vi "De-Initialize.vi"(8 "error in (no error)":errorcluster, 11 "Device in":refnum<class "RS232_Device.lvclass">) -> (0 "error out":errorcluster, 3 "Device out":refnum<class "RS232_Device.lvclass">)   [LabVIEW 2023, in "RS232_Device.lvclass"]
uses:
  RS232_Device.lvclass
  RS232_Device.lvclass/RS232_Device.ctl
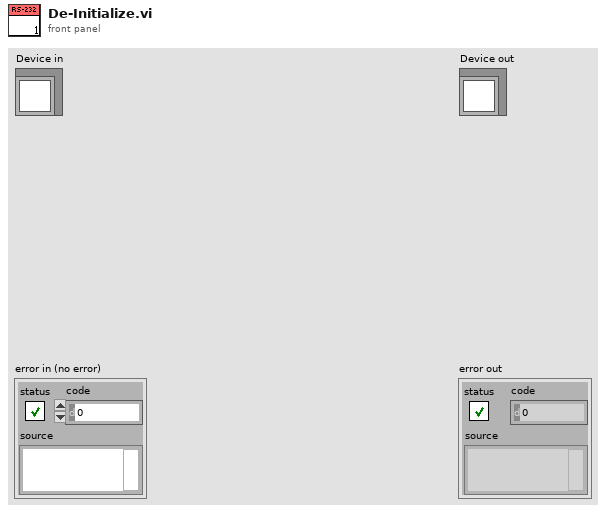
[diagram p1: front panel]
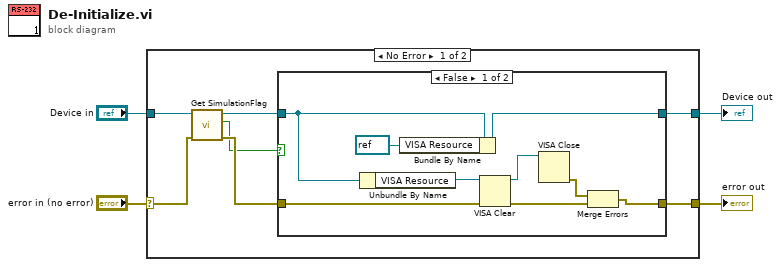
[diagram p0: block diagram]
diagram:
  n1 = case shown="No Error" "error in (no error)" {
    selector: "error in (no error)" -> [w7 w24]
    tunnel: [w11 w24] -> w3
    tunnel: [w10 w23] -> w1
    tunnel: "Device in" -> [w8 w23]
    frame No Error {
      n2 = call-dynamic "Get SimulationFlag.vi"("error in (no error)"=w7, "Device in"=w8) -> ("error out"=w6:errorcluster, "Simulation?"=w5:bool, "Device out"=w9:refnum<class "RS232_Device.lvclass">)  [unwired: 7 in]
      n3 = case shown="False" w5 {
        tunnel: w9 -> [w20 w22]
        tunnel: w6 -> [w15 w21]
        tunnel: [w12 w21] -> w11
        tunnel: [w19 w22] -> w10
        frame False {
          n4 = Unbundle By Name(w20) -> ("VISA Resource"=w17:refnum<visa-resource-name>)
          n5 = Bundle By Name(cluster=w20, "VISA Resource"=refnum<visa-resource-name> refnum) -> (w19:refnum<class "RS232_Device.lvclass">)
          n6 = VISA Clear(VISA resource name=w17, error in (no error)=w15) -> (VISA resource name out=w16:refnum<visa-resource-name>, error out=w13:errorcluster)
          n7 = VISA Close(VISA resource name=w16) -> (error out=w14:errorcluster)  [unwired: 1 in]
          n8 = Merge Errors(w14, w13) -> (w12:errorcluster)
        }
        frame True {
        }
      }
    }
    frame Error {
    }
  }
  "error out" <- w3
  "Device out" <- w1
